vi "Get Text.vi"(8 "Error In":errorcluster, 11 "Pixel In":refnum<class "String.lvclass">) -> (0 "Error Out":errorcluster, 2 "Text":string, 3 "Pixel Out":refnum<class "String.lvclass">)   [LabVIEW 2019, in "String.lvclass"]
uses:
  String.lvclass
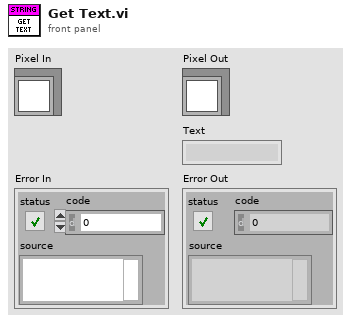
[diagram p1: front panel]
types:
  T1 = typedef "String.lvclass/Data.ctl" = cluster{"Text":string, "Letters Array":void[]}
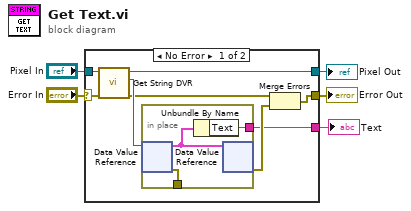
[diagram p0: block diagram]
diagram:
  n1 = case shown="No Error" "Error In" {
    selector: "Error In" -> [w9 w17]
    tunnel: [w11 w17] -> w4
    tunnel: [w7 w18] -> w2
    tunnel: "Pixel In" -> [w10 w18]
    tunnel: [w12 _] -> w1
    frame No Error {
      n2 = call "Get String DVR.vi"("Error In"=w9, "Pixel In"=w10) -> ("Error Out"=w6:errorcluster, "DVR"=w8:refnum<data-value>, "Pixel Out"=w7:refnum<class "String.lvclass">)  [unwired: 7 in]
      n3 = in-place {
        in-place-border: [w14] -> w12
        in-place-border: [w16] -> _
        n4 = in-place-dvr #1(w8) -> (w15:T1, w16:errorcluster)
        n5 = Unbundle By Name(w15) -> ("Text"=w14:string)
        n6 = in-place-dvr #1(w15) -> (w13:errorcluster)  [unwired: 1 out]
      }
      n7 = Merge Errors(w6, w13) -> (w11:errorcluster)
    }
    frame Error {
    }
  }
  "Pixel Out" <- w2
  "Error Out" <- w4
  "Text" <- w1
